vi "Odometry.vi"() -> ()   [LabVIEW 2019]
uses:
  <vilib>/Platform/TimedLoop/XDataNode/timing_clust.ctl
  <vilib>/Platform/TimedLoop/XDataNode/nitl_modes.ctl
  <vilib>/Platform/TimedLoop/XDataNode/wakeup.ctl
  <vilib>/myRIO/Common/Instrument Driver Framework/myRIO v1.0/Encoder/typedefs/Encoder Signal Mode.ctl
  <vilib>/myRIO/Instrument Drivers/Onboard IO/Encoder/typedefs/Encoder Reference.ctl
  <vilib>/myRIO/Common/Instrument Driver Framework/Utilities/typedefs/myRIO Generic Hardware Reference.ctl
  <vilib>/myRIO/Common/Instrument Driver Framework/Utilities/typedefs/Hardware Version Enum.ctl
  <vilib>/myRIO/Common/Instrument Driver Framework/Utilities/typedefs/myRIO v1.0 Reference.ctl
  <vilib>/myRIO/Common/Instrument Driver Framework/Utilities/typedefs/Generic FPGA Reference.ctl
  <vilib>/myRIO/Common/Instrument Driver Framework/myRIO v1.0/Encoder/typedefs/Encoder Channels Enum.ctl
  <vilib>/myRIO/Common/Instrument Driver Framework/myRIO v1.0/Encoder/typedefs/Encoder Configuration v1.0.ctl
  <vilib>/userDefined/High Color/nirio_resource_hc.ctl
  <vilib>/myRIO/Instrument Drivers/Onboard IO/PWM/typedefs/PWM Reference.ctl
  <vilib>/myRIO/Common/Instrument Driver Framework/myRIO v1.0/PWM/typedefs/PWM Channels Enum.ctl
  <vilib>/myRIO/Instrument Drivers/Onboard IO/PWM/typedefs/PWM Configuration.ctl
  <vilib>/myRIO/Instrument Drivers/Onboard IO/DIO/typedefs/DIO Reference.ctl
  <vilib>/myRIO/Common/Instrument Driver Framework/myRIO v1.0/DIO/typedefs/DIO Channels List.ctl
  <vilib>/myRIO/Common/Instrument Driver Framework/myRIO v1.0/DIO/typedefs/DIO Channels Enum.ctl
  <vilib>/myRIO/Common/Instrument Driver Framework/Utilities/vis/Is FPGA Ref Available.vi
  <vilib>/myRIO/Common/Instrument Driver Framework/myRIO v1.0/Encoder/vis/myRIO v1.1 Open Encoder.vi
  <vilib>/myRIO/Instrument Drivers/Onboard IO/Encoder/vis/Read.vi
  <vilib>/myRIO/Common/Instrument Driver Framework/myRIO v1.0/PWM/vis/myRIO v1.1 Open PWM.vi
  <vilib>/myRIO/Instrument Drivers/Onboard IO/PWM/vis/Set Duty Cycle and Frequency.vi
  <vilib>/myRIO/Common/Instrument Driver Framework/myRIO v1.0/DIO/vis/myRIO v1.1 Open DIO.vi
  <vilib>/myRIO/Instrument Drivers/Onboard IO/DIO/vis/Write.vi
  <vilib>/myRIO/Common/Instrument Driver Framework/Utilities/vis/Validate Channels.vi
  <vilib>/myRIO/Common/Instrument Driver Framework/myRIO v1.0/Encoder/vis/myRIO v1.0 Reserve Encoder.vi
  <vilib>/myRIO/Common/Instrument Driver Framework/myRIO v1.0/PWM/vis/myRIO v1.0 Reserve PWM.vi
  <vilib>/myRIO/Common/Instrument Driver Framework/myRIO v1.0/DIO/vis/myRIO v1.0 Reserve DIO.vi
  <vilib>/myRIO/Common/Instrument Driver Framework/myRIO v1.0/Encoder/vis/myRIO v1.0 Build MUX Configuration Encoder.vi
  <vilib>/myRIO/Common/Instrument Driver Framework/myRIO v1.0/Resource Manager/vis/myRIO v1.0 Reserve Channel List.vi
  <vilib>/myRIO/Common/Instrument Driver Framework/myRIO v1.0/PWM/vis/myRIO v1.0 Build MUX Configuration PWM.vi
  <vilib>/myRIO/Common/Instrument Driver Framework/myRIO v1.0/DIO/vis/myRIO v1.0 Build MUX Configuration DIO.vi
  <vilib>/myRIO/Common/Instrument Driver Framework/myRIO v1.0/Resource Manager/vis/myRIO v1.0 Create Configuration List.vi
  <vilib>/myRIO/Common/Instrument Driver Framework/myRIO v1.0/Resource Manager/vis/myRIO v1.0 Reserve Channel.vi
  <vilib>/myRIO/Common/Instrument Driver Framework/myRIO v1.0/Resource Manager/vis/myRIO v1.0 Unreserve Channel.vi
  <vilib>/myRIO/Common/Instrument Driver Framework/myRIO v1.0/Resource Manager/vis/myRIO v1.0 Build Mutex Name.vi
  <vilib>/Utility/VariantDataType/GetNumericInfo.vi
  <vilib>/Utility/error.llb/Error Cluster From Error Code.vi
  <vilib>/myRIO/Common/Instrument Driver Framework/myRIO v1.0/myRIO v1.1 Open.vi
  <vilib>/myRIO/Common/Instrument Driver Framework/Utilities/vis/IO Manager.vi
  <vilib>/myRIO/Common/Instrument Driver Framework/Utilities/vis/Configuration Manager.vi
  <vilib>/myRIO/Common/Instrument Driver Framework/myRIO v1.0/Resource Manager/vis/myRIO v1.0 Configure IO.vi
  <vilib>/myRIO/Common/Instrument Driver Framework/myRIO v1.0/myRIO v1.0 Close.vi
  <vilib>/myRIO/Common/Instrument Driver Framework/myRIO v1.0/Encoder/vis/myRIO v1.0 Configure Encoder.vi
  <vilib>/myRIO/Common/Instrument Driver Framework/myRIO v1.0/Encoder/vis/myRIO v1.0 Read Encoder.vi
  <vilib>/imath/engines/lvmath2/RunTimeEngine/NodeEndStatement/NIMS_NodeEndStatement_Output.vi
  <instcachedir>/0/NIMS_NodeEndStatement_Output_53EC0D466D134D7ABD903AC30B43404B.lvgen/NIMS_NodeEndStatement_Output_53EC0D466D134D7ABD903AC30B43404B_001.vi
  <instcachedir>/0/NIMS_NodeEndStatement_Output_53EC0D466D134D7ABD903AC30B43404B.lvgen/NIMS_NodeEndStatement_Output_53EC0D466D134D7ABD903AC30B43404B_010.vi
  <vilib>/imath/engines/lvmath2/RunTimeEngine/ErrorHandling/NIMS_Finalize Error.vi
  <vilib>/myRIO/Common/Instrument Driver Framework/myRIO v1.0/PWM/vis/myRIO v1.0 Write PWM.vi
  <vilib>/myRIO/Common/Instrument Driver Framework/myRIO v1.0/DIO/vis/myRIO v1.0 Write DIO.vi
  <vilib>/platform/TimedLoop/XDataNode/XDataNode.xnode
  <vilib>/myRIO/Express VI/Onboard IO/Encoder/Encoder Express VI.xnode
  <vilib>/myRIO/Instrument Drivers/Onboard IO/Encoder/vis/myRIO Encoder Open.xnode
  <vilib>/myRIO/Common/Instrument Driver Framework/myRIO v1.0/Encoder/typedefs/Encoder Count Direction Enum.ctl
  <vilib>/myRIO/Express VI/Onboard IO/PWM/PWM Express VI.xnode
  <vilib>/myRIO/Instrument Drivers/Onboard IO/PWM/vis/myRIO PWM Open.xnode
  <vilib>/myRIO/Express VI/Onboard IO/DO/DO Express VI.xnode
  <vilib>/myRIO/Instrument Drivers/Onboard IO/DIO/vis/myRIO DIO Open.xnode
  <vilib>/Platform/TimedLoop/XDataNode/XDNodeRunTimeDep.lvlib
  <vilib>/myRIO/Instrument Drivers/Onboard IO/DIO/DIO.lvlib
  <vilib>/myRIO/Instrument Drivers/Onboard IO/Encoder/Encoder.lvlib
  <vilib>/myRIO/Instrument Drivers/Onboard IO/PWM/PWM.lvlib
panel:
  out "Waveform Chart 4":cluster{"actCarV":dbl, "desCarV":dbl}(graph)
  out "Waveform Chart 3":cluster{"actCarOmega":dbl, "desCarOmega":dbl}(graph)
  out "phi L now, desired":cluster{dbl, "omegaL":dbl}(graph)
  out "phi R now, desired":cluster{dbl, "omegaR":dbl}(graph)
  out "XY Graph":dbl[][](graph)
  out "Duty 3":dbl
  in  "Frequency [Hz] 3":dbl=1000.0
  out "Duty 2":dbl
  in  "Frequency [Hz] 2":dbl=1000.0
  in  "stop 2":bool
  in  "Tab Control":enum32{"Page 1", "Page 2", "Page 3"}(tab)
  in  "t1":dbl
  in  "t2":dbl
  in  "t3":dbl
  in  "Vmax (m/s)":dbl
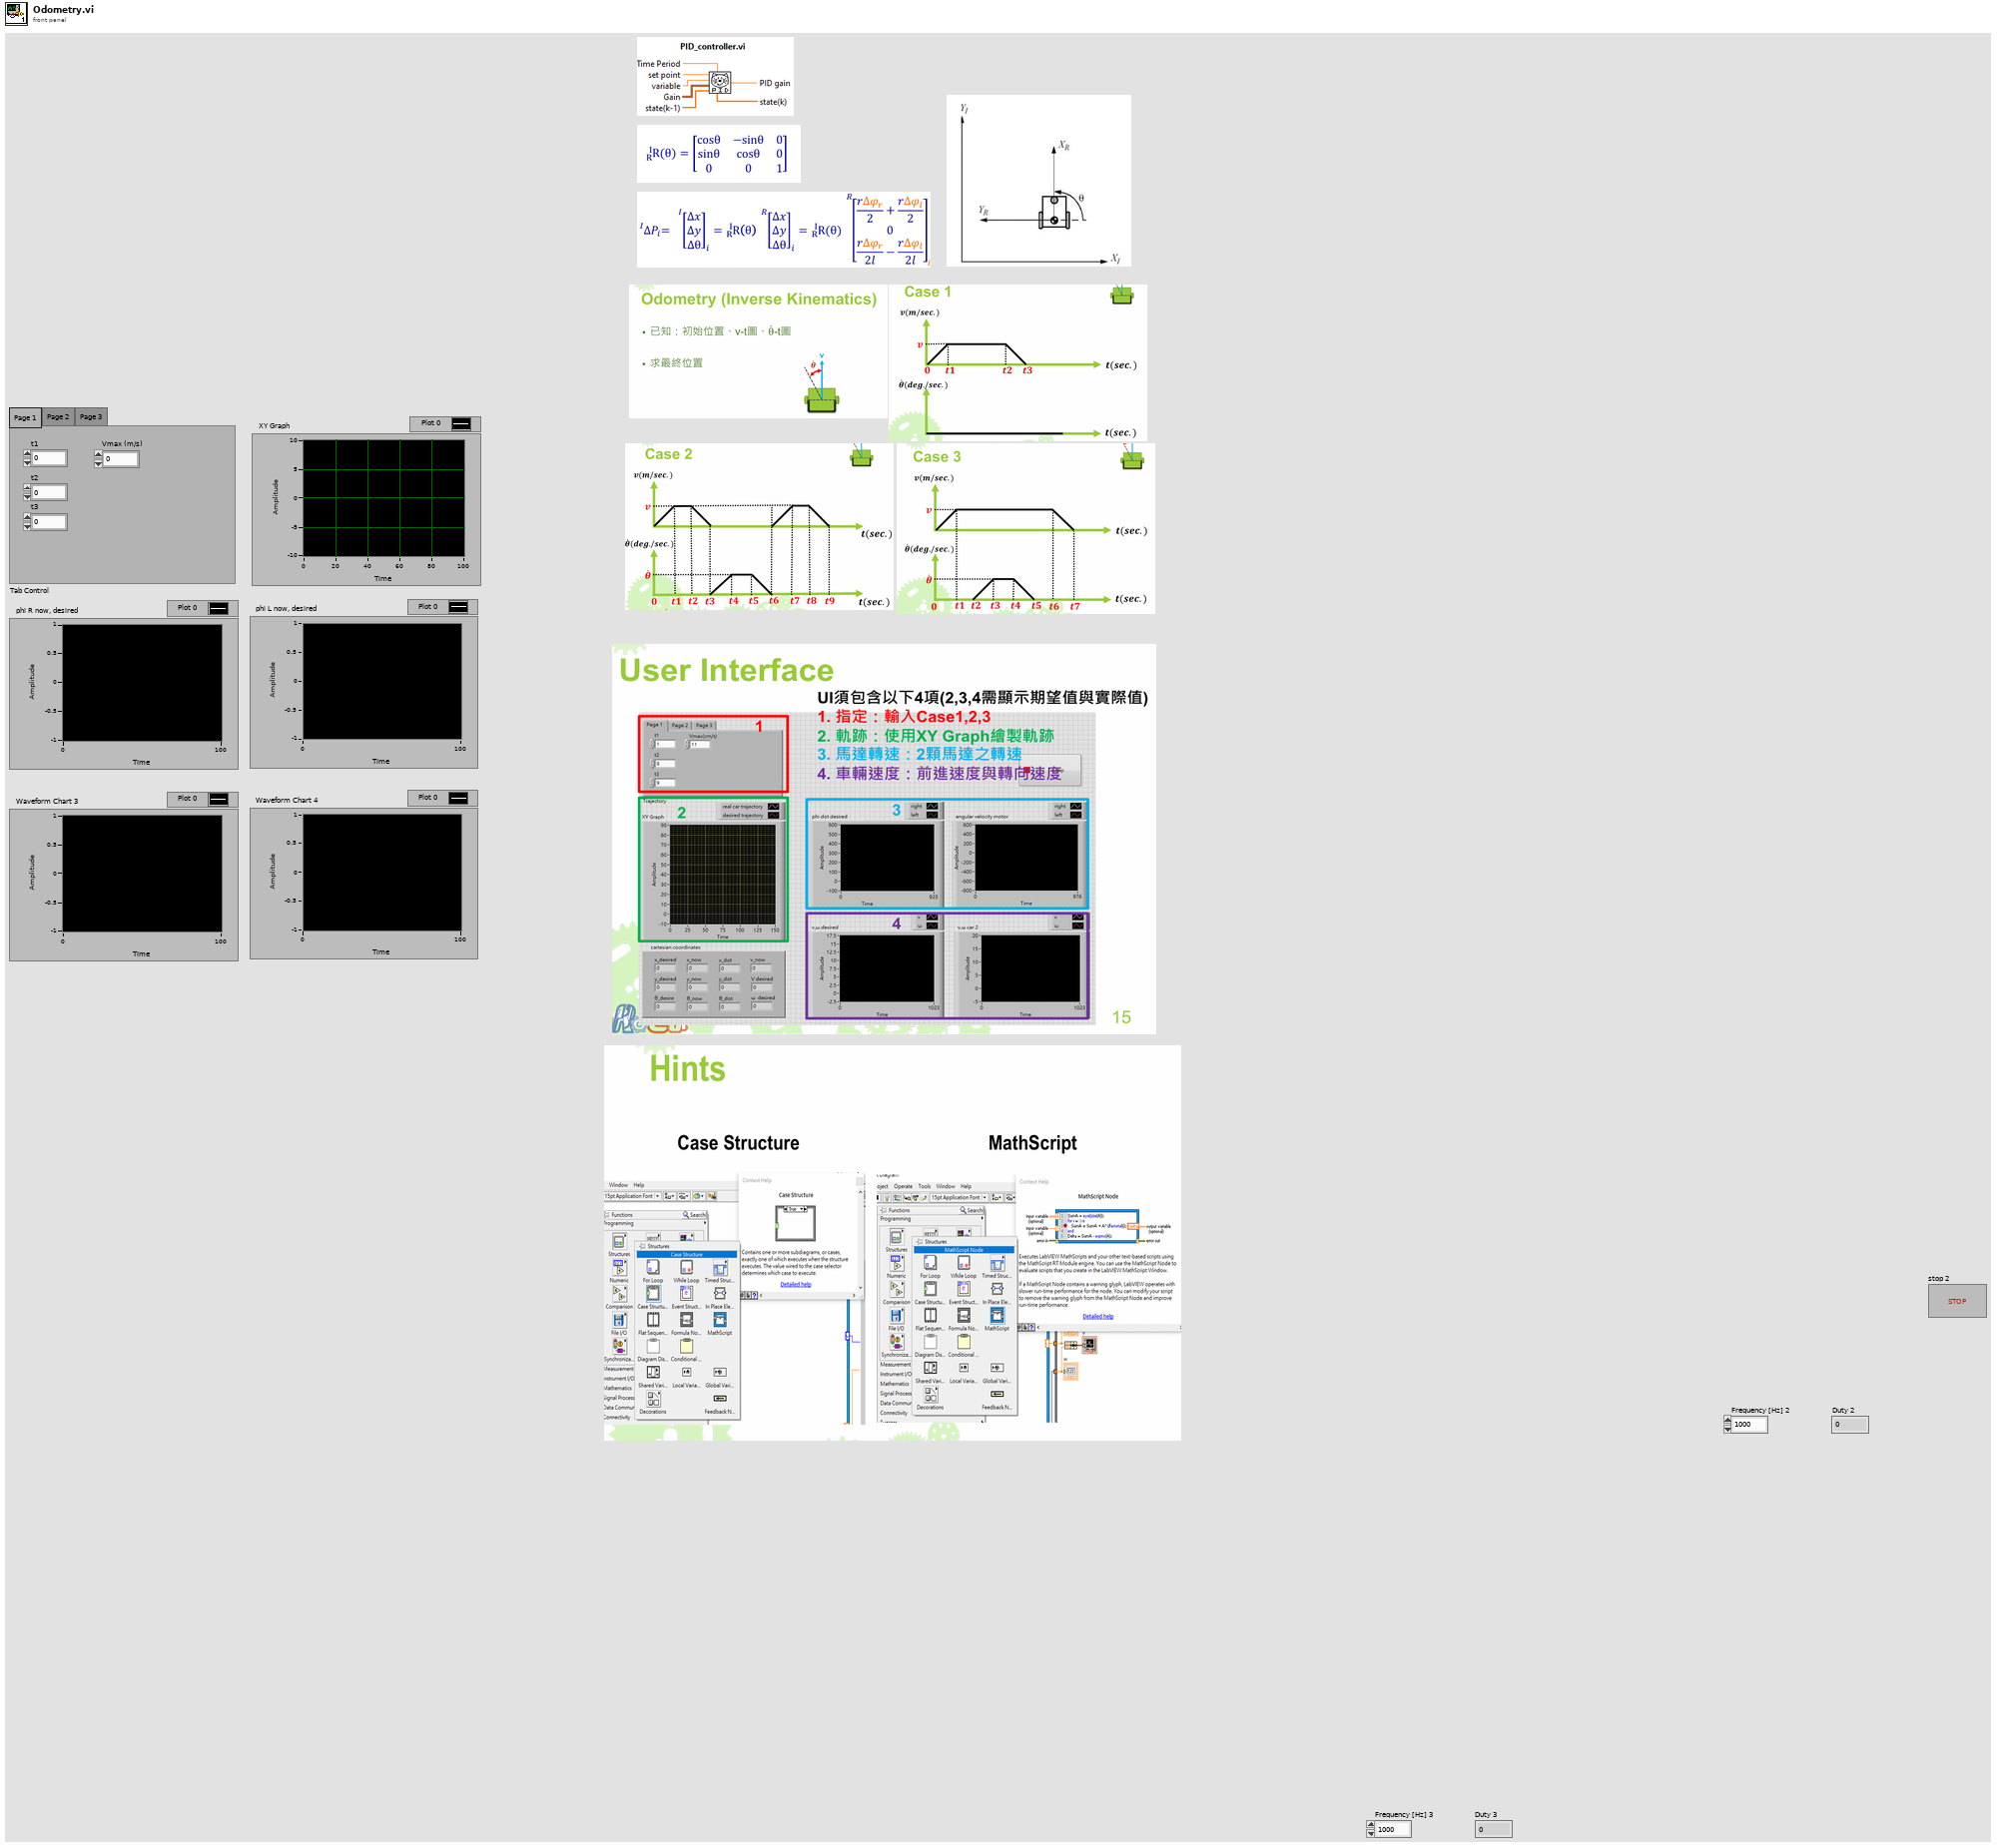
[diagram p1: front panel]
types:
  T1 = typedef "PWM.lvlib/PWM Reference.ctl" = cluster{"myRIO Reference":T2, "PWM Channels Enum":T6, "PWM Configuration":T7}
  T2 = typedef "myRIO Generic Hardware Reference.ctl" = cluster{"myRIO Model":T3, "myRIO Hardware Reference":T4}
  T3 = typedef "Hardware Version Enum.ctl" = enum16{"Unknown", "myRIO-1900", "myRIO-1950", "roboRIO", "NI ELVIS RIO CM", "ELVIS III"}
  T4 = typedef "myRIO v1.0 Reference.ctl" = cluster{"Generic FPGA Reference":T5, "Allow multiple opens":bool}
  T5 = typedef "Generic FPGA Reference.ctl" = refnum<k20>
  T6 = typedef "PWM Channels Enum.ctl" = enum16{"Not Connected", "C/PWM0", "C/PWM1", "A/PWM0", "A/PWM1", "A/PWM2", "A/PWM3", "A/PWM4", "A/PWM5", "A/PWM6", "A/PWM7", "A/PWM8", "A/PWM9", "A/PWM10", "A/PWM11", "A/PWM12", "A/PWM13", "A/PWM14", "A/PWM15", "A/PWM16", "A/PWM17", "A/PWM18", "A/PWM19", "B/PWM0", "B/PWM1", "B/PWM2", "B/PWM3", "B/PWM4", "B/PWM5", "B/PWM6", "B/PWM7", "B/PWM8", "B/PWM9", "B/PWM10", "B/PWM11", "B/PWM12", "B/PWM13", "B/PWM14", "B/PWM15", "B/PWM16", "B/PWM17", "B/PWM18", "B/PWM19", "PWM/PWM0", "PWM/PWM1", "PWM/PWM2", "PWM/PWM3", "PWM/PWM4", "PWM/PWM5", "PWM/PWM6", "PWM/PWM7", "PWM/PWM8", "PWM/PWM9"}
  T7 = typedef "PWM.lvlib/PWM Configuration.ctl" = cluster{"Frequency":dbl, "Duty Cycle":dbl}
  T8 = typedef "nirio_resource_hc.ctl" = tag
  T9 = typedef "DIO.lvlib/DIO Reference.ctl" = cluster{"myRIO Reference":T2, "DIO Channels List":T10}
  T10 = typedef "DIO Channels List.ctl" = T11[]
  T11 = typedef "DIO Channels Enum.ctl" = enum16{"Not Connected", "C/DIO0", "C/DIO1", "C/DIO2", "C/DIO3", "C/DIO4", "C/DIO5", "C/DIO6", "C/DIO7", "A/DIO0", "A/DIO1", "A/DIO2", "A/DIO3", "A/DIO4", "A/DIO5", "A/DIO6", "A/DIO7", "A/DIO8", "A/DIO9", "A/DIO10", "A/DIO11", "A/DIO12", "A/DIO13", "A/DIO14", "A/DIO15", "A/DIO16", "A/DIO17", "A/DIO18", "A/DIO19", "B/DIO0", "B/DIO1", "B/DIO2", "B/DIO3", "B/DIO4", "B/DIO5", "B/DIO6", "B/DIO7", "B/DIO8", "B/DIO9", "B/DIO10", "B/DIO11", "B/DIO12", "B/DIO13", "B/DIO14", "B/DIO15", "B/DIO16", "B/DIO17", "B/DIO18", "B/DIO19", "LED0", "LED1", "LED2", "LED3", "Button0", "DIO/DIO0", "DIO/DIO1", "DIO/DIO2", "DIO/DIO3", "DIO/DIO4", "DIO/DIO5", "DIO/DIO6", "DIO/DIO7", "DIO/DIO8", "DIO/DIO9", "SPI/CS0", "SPI/CS1", "SPI/CS2", "SPI/CS3", "LED RADIO (Green)", "LED RADIO (Red)", "LED COMM (Green)", "LED COMM (Red)", "LED MODE (Green)", "LED MODE (Red)"}
  T12 = typedef "Encoder.lvlib/Encoder Reference.ctl" = cluster{"myRIO Reference":T2, "Encoder Channels Enum":T13}
  T13 = typedef "Encoder Channels Enum.ctl" = enum16{"Not Connected", "C/ENC0", "C/ENC1", "A/ENC", "A/ENC0", "A/ENC1", "A/ENC2", "A/ENC3", "A/ENC4", "A/ENC5", "A/ENC6", "A/ENC7", "A/ENC8", "A/ENC9", "B/ENC", "B/ENC0", "B/ENC1", "B/ENC2", "B/ENC3", "B/ENC4", "B/ENC5", "B/ENC6", "B/ENC7", "B/ENC8", "B/ENC9", "DIO/ENC0", "DIO/ENC1", "DIO/ENC2", "DIO/ENC3", "DIO/ENC4"}
  T14 = typedef "Encoder Signal Mode.ctl" = enum16{"Quadrature phase signal", "Step and direction signal"}
  T15 = typedef "XDNodeRunTimeDep.lvlib/timing_clust.ctl" = cluster{"Expected End [f-1]":u64, "Actual End [f-1]":u64, "Finished Late? [f-1]":bool, "Expected End [i-1]":u64, "Actual End [i-1]":u64, "Finished Late? [i-1]":bool, "Expected Start [i]":u64, "Actual Start [i]":u64, "Expected Start [f]":u64, "Actual Start [f]":u64, "Source Name":string, "Structure Name":string, "Period":i64, "Deadline":i64, "Offset":i64, "Start":i64, "Priority":i32, "Timeout":i32, "Mode":T16, "Wakeup Reason":T17, "Error":errorcluster, "Source Type":string, "Secondary Source Type":string, "Global End Time":u64, "Global Start Time":u64, "Frame Duration":u64, "Iteration Duration":u64, "Assigned CPU":i32, "I/O Scan Engine Mode":u32}
  T16 = typedef "XDNodeRunTimeDep.lvlib/nitl_modes.ctl" = enum32{"No Change", "Process missed periods, maintain original phase", "Discard missed periods, maintain original phase", "Process missed periods, ignore original phase", "Discard missed periods, ignore original phase"}
  T17 = typedef "XDNodeRunTimeDep.lvlib/wakeup.ctl" = enum32{"Normal", "Aborted", "Asynchronous wakeup", "Timing source error", "Timed loop error", "Timeout"}
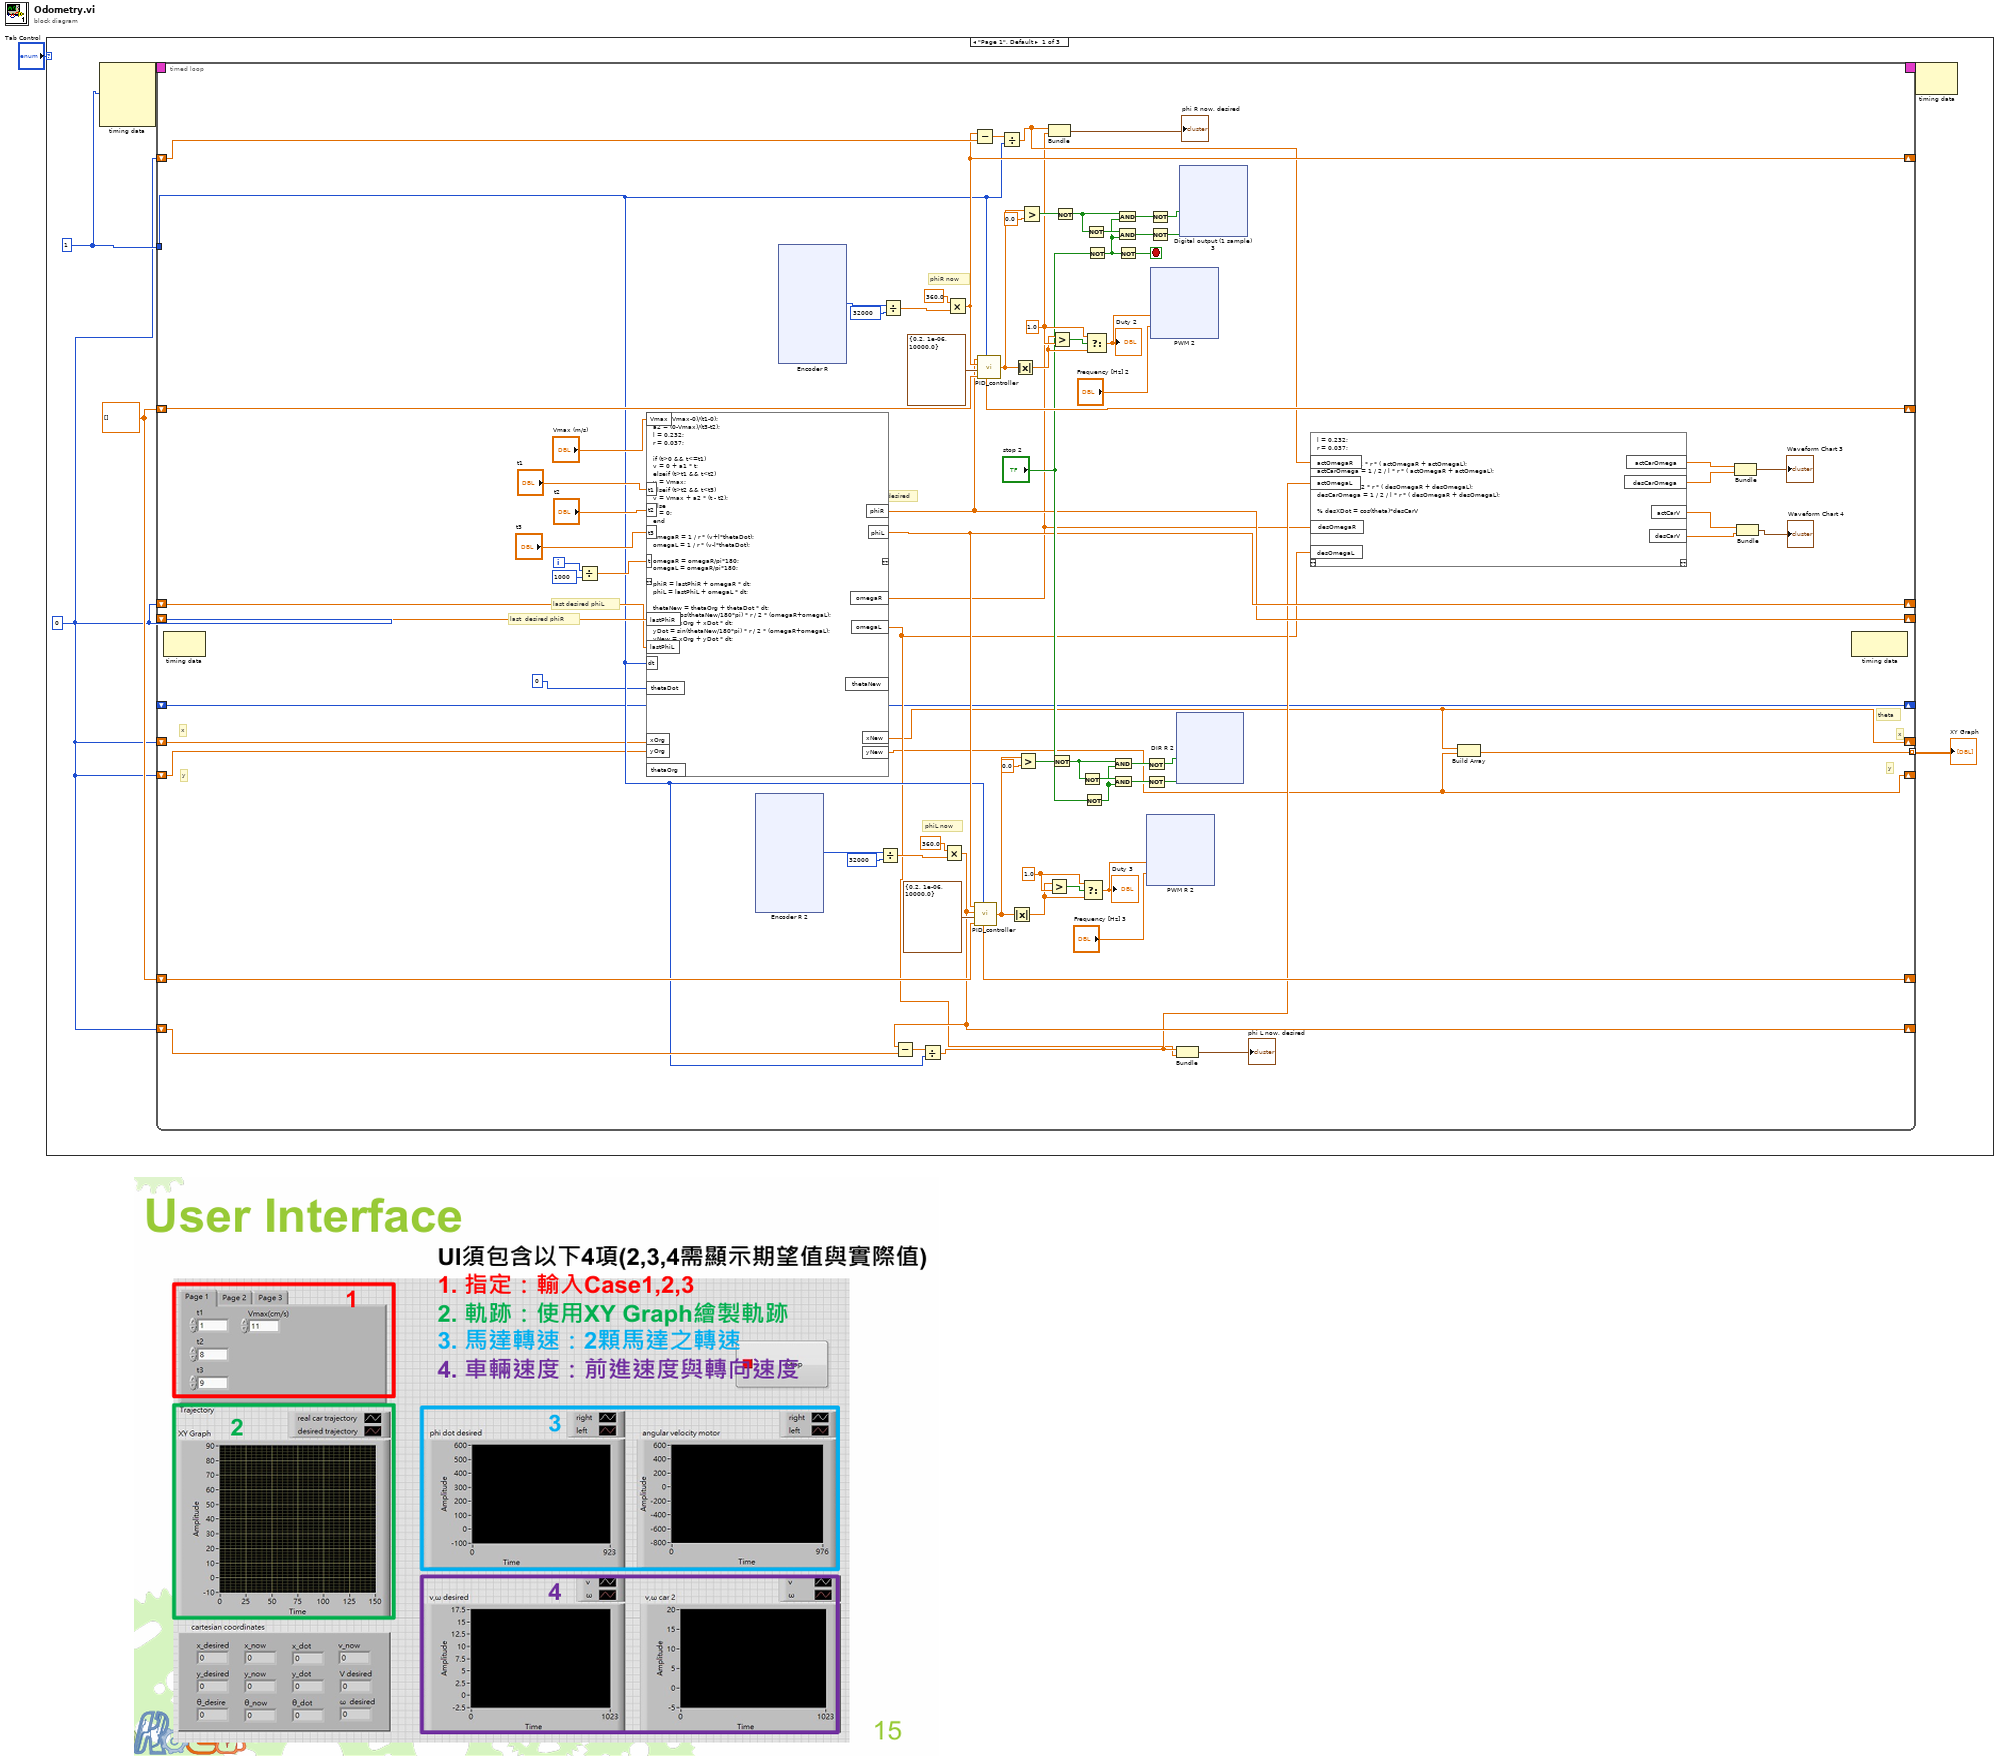
[diagram p0: block diagram]
diagram:
  n1 = case shown="\"Page 1\", Default" "Tab Control" {
    frame "Page 1", Default {
      w5 = dbl[] [] ("state(k)")
      w3 = 0
      w4 = i64 1 ("Period")
      n2 = node-c288(w4) -> (w7:T15)  [unwired: 3 in]
      n3 = timed-loop {
        timing: w7 -> [_]
        timing-out: [_] -> w6
        shift-right: [w31] -> _
        shift-left: w3 -> [w85]
        shift-right: [w32] -> _
        shift-left: w3 -> [w84]
        tunnel: w4 -> [w27]
        shift-right: [w77] -> _
        shift-left: w5 -> [w78]
        shift-right: [w39] -> _
        shift-left: w5 -> [w38]
        shift-right: [w35] -> _
        shift-left: w3 -> [w36]
        shift-right: [w28] -> _
        shift-left: w3 -> [w29]
        shift-right: [w14] -> _
        shift-left: _ -> [w13]
        shift-right: [w10] -> _
        shift-left: w3 -> [w12]
        shift-right: [w9] -> _
        shift-left: w3 -> [w11]
        tunnel: [w8] -> w2 mode=indexing
        i -> [w88]
        stop <- w67 stop-if-true
        w43 = 1.0 ("y")
        w64 = 1.0 ("y")
        # "y"
        # "y"
        # "x"
        # "x"
        # "theta"
        # "desired"
        # "phiL now"
        # "phiR now"
        # "last desired phiL"
        # "last  desired phiR"
        n4 = node-c288() -> ()  [unwired: 1 in, 1 out]
        n5 = Divide(x=w88, y=1000) -> (x/y=w86:dbl)
        n6 = mathscript code="a1 = (Vmax-0)/(t1-0);\na2 = (0-Vmax)/(t3-t2);\nl = 0.232;\nr = 0.037;\n\nif (t>0 && t<=t1)\nv = 0 + a1 * t;\nelseif (t>t1 && t<t2)\nv = Vmax;\nelseif (t>t2 && t<t3)\nv = Vmax + a2 * (t - t2);\nelse\nv = 0;\nend\n\nomegaR = 1 / r * (v+l*thetaDot);\nomegaL = 1 / r * (v-l*thetaDot);\n\nomegaR = omegaR/pi*180;\nomegaL = omegaR/pi*180;\n\nphiR = lastPhiR + omegaR * dt;\nphiL = lastPhiL + omegaL * dt;\n\nthetaNew = thetaOrg + thetaDot * dt;\nxDot = cos(thetaNew/180*pi) * r / 2 * (omegaR+omegaL);\nxNew = xOrg + xDot * dt;\nyDot = sin(thetaNew/180*pi) * r / 2 * (omegaR+omegaL);\nyNew = xOrg + yDot * dt;"("t1"="t1", "t2"="t2", "t3"="t3", "Vmax"="Vmax (m/s)", "t"=w86, "lastPhiR"=w85, "lastPhiL"=w84, "dt"=w27, "thetaDot"=0, "thetaOrg"=w13, "xOrg"=w12, "yOrg"=w11) -> ("omegaR"=w23:dbl, "omegaL"=w22:dbl, "phiL"=w32:dbl, "phiR"=w31:dbl, "thetaNew"=w14:i64, "xNew"=w10:dbl, "yNew"=w9:dbl)  [unwired: 1 in, 1 out]
        n7 = xnode "Encoder R 2"() -> ("Counter Value"=w58:i32)  [unwired: 2 in, 3 out]
        n8 = xnode "Encoder R"() -> ("Counter Value"=w82:i32)  [unwired: 2 in, 3 out]
        n9 = Divide(x=w58, y=32000) -> (x/y=w59:dbl)
        n10 = Divide(x=w82, y=32000) -> (x/y=w83:dbl)
        n11 = Multiply(x=360.0, y=w59) -> (x*y=w28:dbl)
        n12 = Subtract(x=w28, y=w29) -> (x-y=w30:dbl)
        n13 = Divide(x=w30, y=w27) -> (x/y=w24:dbl)
        n14 = Multiply(x=360.0, y=w83) -> (x*y=w35:dbl)
        n15 = Subtract(x=w35, y=w36) -> (x-y=w34:dbl)
        n16 = call "PID_controller.vi"("Time Period"=w27, "state(k-1)"=w38, "Gain"=cluster{dbl, dbl, dbl} {0.2, 1e-06, 10000.0}, "variable"=w28, "set point"=w32) -> ("PID gain"=w41:dbl, "state(k)"=w39:dbl[])
        n17 = call "PID_controller.vi"("Time Period"=w27, "state(k-1)"=w78, "Gain"=cluster{dbl, dbl, dbl} {0.2, 1e-06, 10000.0}, "variable"=w35, "set point"=w31) -> ("PID gain"=w62:dbl, "state(k)"=w77:dbl[])
        n18 = Divide(x=w34, y=w27) -> (x/y=w25:dbl)
        n19 = Absolute Value(x=w41) -> (abs(x)=w42:dbl)
        n20 = Absolute Value(x=w62) -> (abs(x)=w63:dbl)
        n21 = Greater?(x=w41, y=0.0) -> (0:w49:bool)
        n22 = Greater?(x=w62, y=0.0) -> (0:w71:bool)
        n23 = Greater?(x=w42, y=w43) -> (0:w44:bool)
        n24 = Bundle(w25, "omegaR"=w23) -> (→"phi R now, desired":cluster{dbl, "omegaR":dbl})  [unwired: 1 in]
        n25 = Not(x=w49) -> (.not. x?=w50:bool)
        n26 = Greater?(x=w63, y=w64) -> (0:w65:bool)
        n27 = Not(x=w71) -> (.not. x?=w72:bool)
        n28 = Not(x=w50) -> (.not. x?=w47:bool)
        n29 = Select(t=w43, s=w44, f=w42) -> (s? t:f=w40:dbl)
        "Duty 3" <- w40
        n30 = Not(x="stop 2") -> (.not. x?=w46:bool)
        n31 = Not(x=w72) -> (.not. x?=w69:bool)
        n32 = Select(t=w64, s=w65, f=w63) -> (s? t:f=w61:dbl)
        "Duty 2" <- w61
        n33 = Not(x="stop 2") -> (.not. x?=w68:bool)
        n34 = And(x=w50, y=w46) -> (x .and. y?=w53:bool)
        n35 = And(x=w47, y=w46) -> (x .and. y?=w51:bool)
        n36 = And(x=w72, y=w68) -> (x .and. y?=w75:bool)
        n37 = And(x=w69, y=w68) -> (x .and. y?=w73:bool)
        n38 = Not(x=w68) -> (.not. x?=w67:bool)
        n39 = Not(x=w53) -> (.not. x?=w54:bool)
        n40 = Not(x=w51) -> (.not. x?=w52:bool)
        n41 = xnode "PWM R 2"("Duty Cycle"=w40, "Frequency [Hz]"="Frequency [Hz] 3") -> ()  [unwired: 1 in, 1 out]
        n42 = Not(x=w75) -> (.not. x?=w76:bool)
        n43 = Not(x=w73) -> (.not. x?=w74:bool)
        n44 = xnode "PWM 2"("Duty Cycle"=w61, "Frequency [Hz]"="Frequency [Hz] 2") -> ()  [unwired: 1 in, 1 out]
        n45 = xnode "DIR R 2"("A/DIO0 (Pin 11)"=w54, "A/DIO1 (Pin 13)"=w52) -> ()  [unwired: 1 in, 1 out]
        n46 = Bundle(w24, "omegaL"=w22) -> (→"phi L now, desired":cluster{dbl, "omegaL":dbl})  [unwired: 1 in]
        n47 = xnode "Digital output (1 sample) 3"("A/DIO0 (Pin 11)"=w76, "A/DIO1 (Pin 13)"=w74) -> ()  [unwired: 1 in, 1 out]
        n48 = mathscript code="l = 0.232;\nr = 0.037;\n\nactCarV = 1 / 2 * r * ( actOmegaR + actOmegaL);\nactCarOmega = 1 / 2 / l * r * ( actOmegaR + actOmegaL);\n\ndesCarV = 1 / 2 * r * ( desOmegaR + desOmegaL);\ndesCarOmega = 1 / 2 / l * r * ( desOmegaR + desOmegaL);\n\n% desXDot = cos(theta)*desCarV"("desOmegaR"=w23, "desOmegaL"=w22, "actOmegaR"=w25, "actOmegaL"=w24) -> ("actCarOmega"=w21:dbl, "desCarOmega"=w20:dbl, "actCarV"=w18:dbl, "desCarV"=w17:dbl)  [unwired: 1 in, 1 out]
        n49 = Build Array(w10, w9) -> (w8:dbl[])
        n50 = Bundle("actCarOmega"=w21, "desCarOmega"=w20) -> (→"Waveform Chart 3":cluster{"actCarOmega":dbl, "desCarOmega":dbl})  [unwired: 1 in]
        n51 = Bundle("actCarV"=w18, "desCarV"=w17) -> (→"Waveform Chart 4":cluster{"actCarV":dbl, "desCarV":dbl})  [unwired: 1 in]
        n52 = node-c288() -> ()  [unwired: 1 in, 1 out]
      }
      "XY Graph" <- w2
      n53 = node-c288(w6) -> ()  [unwired: 1 out]
    }
    frame "Page 2" {
    }
    frame "Page 3" {
    }
  }
